vi "Where.vi"(6 "TypeMap in":refnum<class "TypeMap.lvclass">, 8 "error in (no error)":errorcluster, 10 "Where in":string[](array[string])) -> (0 "error out":errorcluster, 4 "TypeMap out":refnum<class "TypeMap.lvclass">)   [LabVIEW 2020, in "ORM.lvlib" / "TypeMap.lvclass"]
uses:
  TypeMap.lvclass
  TypeMap.lvclass/TypeMap.ctl
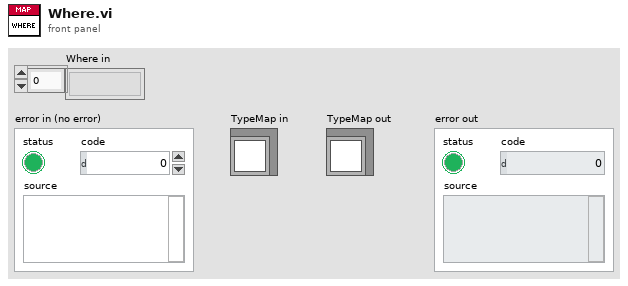
[diagram p1: front panel]
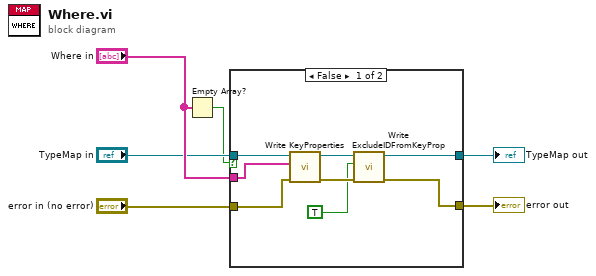
[diagram p0: block diagram]
diagram:
  n1 = Empty Array?(array="Where in") -> (empty?=w1:bool)
  n2 = case shown="False" w1 {
    tunnel: "TypeMap in" -> [w13 w16]
    tunnel: [w12 w16] -> w3
    tunnel: [w9 w15] -> w4
    tunnel: "error in (no error)" -> [w8 w15]
    tunnel: "Where in" -> [w7 _]
    frame False {
      n3 = call "Write KeyProperties.vi"("error in (no error)"=w8, "Key Properties"=w7, "TypeMap in"=w13) -> ("error out"=w14:errorcluster, "TypeMap out"=w11:refnum<class "TypeMap.lvclass">)  [unwired: 7 in]
      n4 = call "Write ExcludeIDFromKeyProp.vi"("error in (no error)"=w14, "ExcludeIDFromKeyProp"=TRUE, "TypeMap in"=w11) -> ("error out"=w9:errorcluster, "TypeMap out"=w12:refnum<class "TypeMap.lvclass">)  [unwired: 7 in]
    }
    frame True {
    }
  }
  "error out" <- w4
  "TypeMap out" <- w3
